vi "Time.vi"(10 "Reset":bool, 11 "Time_Limit":i32) -> (3 "Time_Met":bool)   [LabVIEW 2016, in "ArgoBotLib.lvlib"]
uses:
  ArgoBotLib.lvlib
panel:
  out "Numeric":dbl
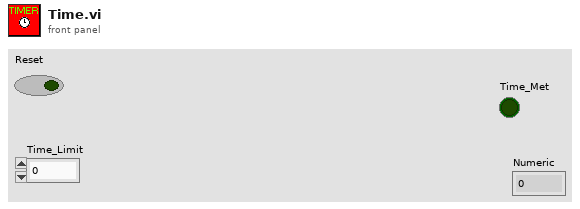
[diagram p1: front panel]
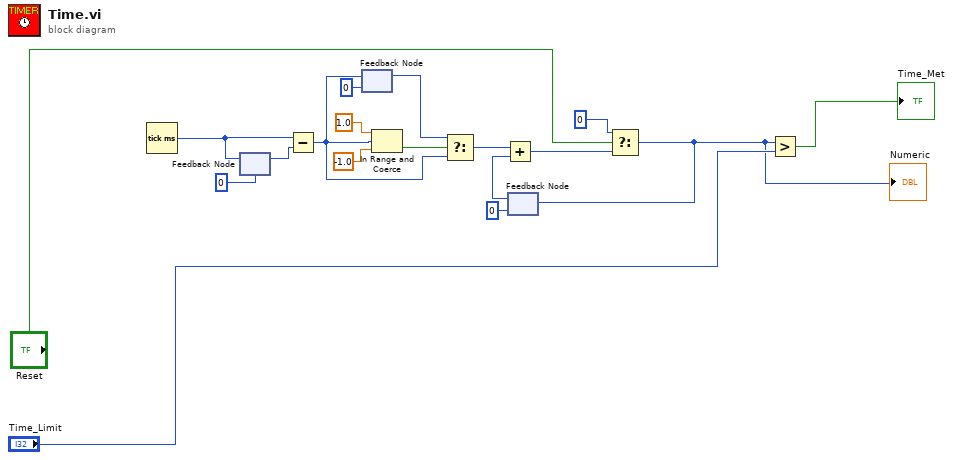
[diagram p0: block diagram]
diagram:
  n1 = Tick Count (ms)() -> (millisecond timer value=w18:u32)
  n2 = feedback #1(u32 0) -> (w17:u32)
  n3 = feedback-in #1(w18) -> ()
  n4 = Subtract(x=w18, y=w17) -> (x-y=w12:u32)
  n5 = feedback #2(u32 0) -> (w13:u32)
  n6 = feedback-in #2(w12) -> ()
  n7 = In Range and Coerce(upper limit=1.0, x=w12, lower limit=-1.0 ("upper limit")) -> (In Range?=w14:bool)  [unwired: 1 out]
  n8 = Select(t=w13, s=w14, f=w12) -> (s? t:f=w11:u32)
  n9 = feedback #3(u32 0) -> (w9:u32)
  n10 = Add(x=w11, y=w9) -> (x+y=w8:u32)
  n11 = Select(t=0, s="Reset", f=w8) -> (s? t:f=w5:u32)
  "Numeric" <- w5
  n12 = feedback-in #3(w5) -> ()
  n13 = Greater?(x=w5, y="Time_Limit") -> (0:→"Time_Met":bool)
